vi "subCreateStagingPaths.vi"(0 "TestStand Version String":string="[2014, 2016, 2017]", 11 "error in":errorcluster) -> (3 "GACUtilityPaths":path[](array[path])=[path "C:/Users/admin/Documents/github/NIVeristandAdd-ons/VeriStand-steps-for-TestStand/Source/Source/CSharp/AddRemoveGACUtils/RemoveFromGAC.exe", path "C:/Users/admin/Documents/github/NIVeristandAdd-ons/VeriStand-steps-for-TestStand/Source/Source/CSharp/AddRemoveGACUtils/InstallToGAC.exe"], 4 "CSharp Assembly Project Path":path=path "C:/Users/admin/Documents/github/NIVeristandAdd-ons/VeriStand-steps-for-TestStand/Source/Source/CSharp/VeristandStepsAssembly/OpenWorkspaceDialog/VeristandSteps.csproj", 6 "TypePalette File Path":path=path "C:/Users/admin/Documents/github/NIVeristandAdd-ons/VeriStand-steps-for-TestStand/Source/Source/CustomPaletteFile/NI_VeristandTypes.ini", 8 "Program Files Destination Path":path=path "C:/Users/admin/Documents/github/NIVeristandAdd-ons/VeriStand-steps-for-TestStand/Source/Built/ProgramFiles_32/VeriStand Steps for TestStand", 10 "Icon File Path":path=path "C:/Users/admin/Documents/github/NIVeristandAdd-ons/VeriStand-steps-for-TestStand/Source/Source/CustomPaletteFile/Veristand_icon_vista.ico", 13 "Icon Paths":path[](array[path])=[path "C:/Users/admin/Documents/github/NIVeristandAdd-ons/VeriStand-steps-for-TestStand/Source/Built/documents/National Instruments/TestStand 2014 (32-bit)/Components/Icons", path "C:/Users/admin/Documents/github/NIVeristandAdd-ons/VeriStand-steps-for-TestStand/Source/Built/documents/National Instruments/TestStand 2014 (64-bit)/Components/Icons", path "C:/Users/admin/Documents/github/NIVeristandAdd-ons/VeriStand-steps-for-TestStand/Source/Built/documents/National Instruments/TestStand 2016 (32-bit)/Components/Icons", path "C:/Users/admin/Documents/github/NIVeristandAdd-ons/VeriStand-steps-for-TestStand/Source/Built/documents/National Instruments/TestStand 2016 (64-bit)/Components/Icons", path "C:/Users/admin/Documents/github/NIVeristandAdd-ons/VeriStand-steps-for-TestStand/Source/Built/documents/National Instruments/TestStand 2017 (32-bit)/Components/Icons", path "C:/Users/admin/Documents/github/NIVeristandAdd-ons/VeriStand-steps-for-TestStand/Source/Built/documents/National Instruments/TestStand 2017 (64-bit)/Components/Icons"], 14 "TypePalettes Paths":path[](array[path])=[path "C:/Users/admin/Documents/github/NIVeristandAdd-ons/VeriStand-steps-for-TestStand/Source/Built/documents/National Instruments/TestStand 2014 (32-bit)/Components/TypePalettes", path "C:/Users/admin/Documents/github/NIVeristandAdd-ons/VeriStand-steps-for-TestStand/Source/Built/documents/National Instruments/TestStand 2014 (64-bit)/Components/TypePalettes", path "C:/Users/admin/Documents/github/NIVeristandAdd-ons/VeriStand-steps-for-TestStand/Source/Built/documents/National Instruments/TestStand 2016 (32-bit)/Components/TypePalettes", path "C:/Users/admin/Documents/github/NIVeristandAdd-ons/VeriStand-steps-for-TestStand/Source/Built/documents/National Instruments/TestStand 2016 (64-bit)/Components/TypePalettes", path "C:/Users/admin/Documents/github/NIVeristandAdd-ons/VeriStand-steps-for-TestStand/Source/Built/documents/National Instruments/TestStand 2017 (32-bit)/Components/TypePalettes", path "C:/Users/admin/Documents/github/NIVeristandAdd-ons/VeriStand-steps-for-TestStand/Source/Built/documents/National Instruments/TestStand 2017 (64-bit)/Components/TypePalettes"], 15 "Error out":errorcluster)   [LabVIEW 2015]
uses:
  veristand-steps-build-tools.lvlib
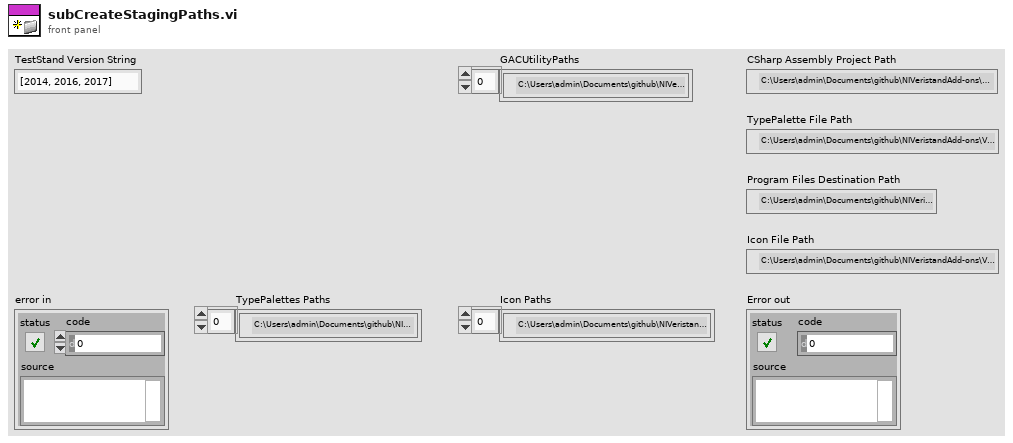
[diagram p1: front panel]
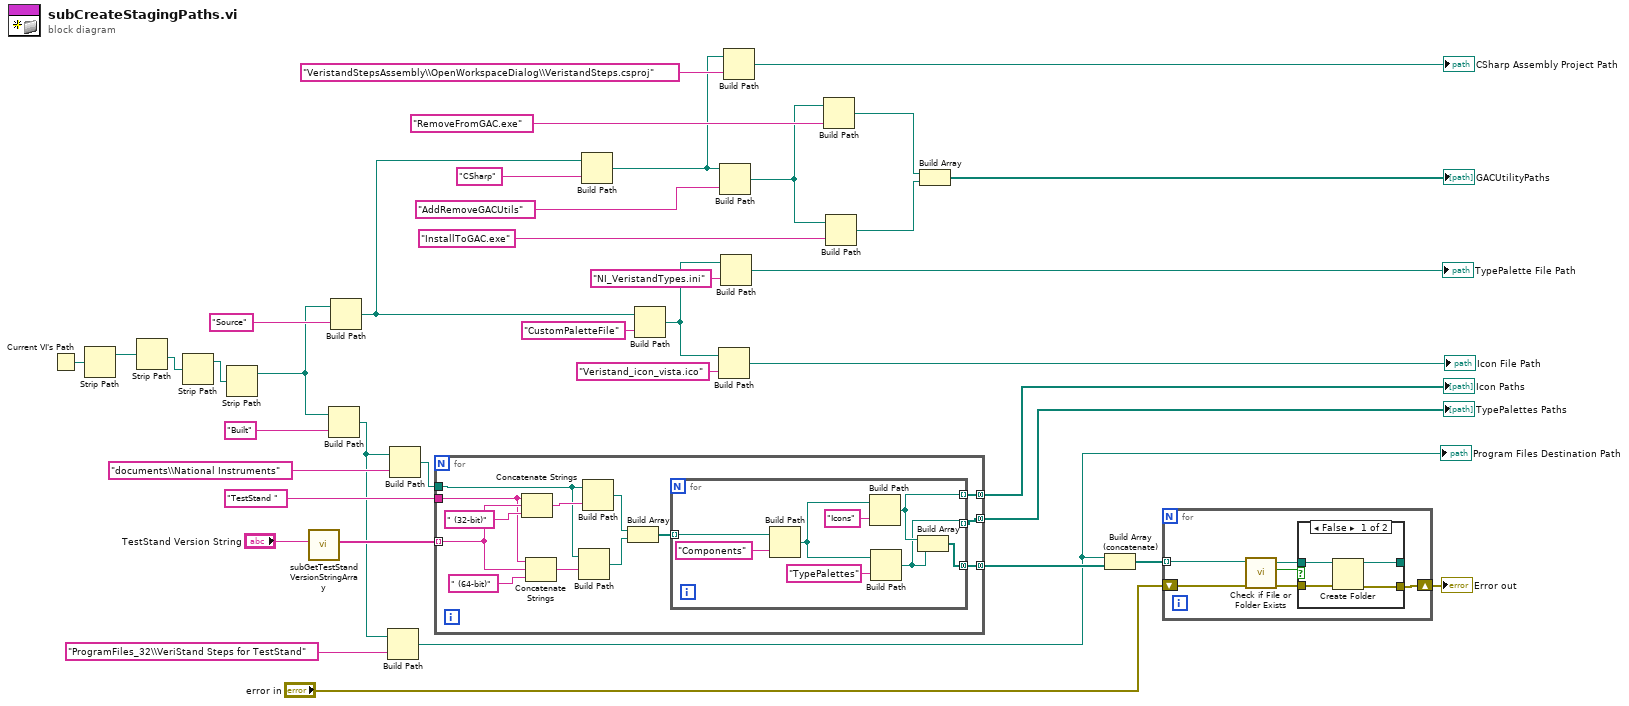
[diagram p0: block diagram]
diagram:
  n1 = Current VI's Path() -> (path=w31:path)
  n2 = Strip Path(path=w31) -> (stripped path=w30:path)  [unwired: 1 out]
  n3 = Strip Path(path=w30) -> (stripped path=w29:path)  [unwired: 1 out]
  n4 = Strip Path(path=w29) -> (stripped path=w2:path)  [unwired: 1 out]
  n5 = Strip Path(path=w2) -> (stripped path=w1:path)  [unwired: 1 out]
  n6 = call "subGetTestStandVersionStringArray.vi"("TestStand Version String"="TestStand Version String") -> ("TestStand Version String Array"=w37:string[])  [unwired: 10 in]
  n7 = Build Path(base path=w1, name or relative path="Built") -> (appended path=w28:path)
  n8 = Build Path(base path=w1, name or relative path="Source") -> (appended path=w11:path)
  n9 = Build Path(base path=w28, name or relative path="ProgramFiles_32\\VeriStand Steps for TestStand") -> (appended path=w13:path)
  "Program Files Destination Path" <- w13
  n10 = Build Path(base path=w28, name or relative path="documents\\National Instruments") -> (appended path=w14:path)
  n11 = for {
    tunnel: w37 -> [w50] mode=indexing
    tunnel: w14 -> [w47]
    tunnel: "TestStand " ("name or relative path") -> [w46]
    tunnel: [w42] -> w32 mode=concatenating
    tunnel: [w41] -> w19 mode=concatenating
    tunnel: [w40] -> w18 mode=concatenating
    n12 = Concatenate Strings(w46, w50, " (32-bit)" ("string")) -> (w48:string)
    n13 = Concatenate Strings(w46, w50, " (64-bit)" ("string")) -> (w49:string)
    n14 = Build Path(base path=w47, name or relative path=w49) -> (appended path=w44:path)
    n15 = Build Path(base path=w47, name or relative path=w48) -> (appended path=w45:path)
    n16 = Build Array(w45, w44) -> (w43:path[])
    n17 = for {
      tunnel: w43 -> [w60] mode=indexing
      tunnel: [w55] -> w42 mode=concatenating
      tunnel: [w54] -> w41 mode=indexing
      tunnel: [w53] -> w40 mode=indexing
      n18 = Build Path(base path=w60, name or relative path="Components") -> (appended path=w57:path)
      n19 = Build Path(base path=w57, name or relative path="Icons") -> (appended path=w54:path)
      n20 = Build Path(base path=w57, name or relative path="TypePalettes") -> (appended path=w53:path)
      n21 = Build Array(w54, w53) -> (w55:path[])
    }
  }
  "Icon Paths" <- w19
  "TypePalettes Paths" <- w18
  n22 = Build Path(base path=w11, name or relative path="CSharp") -> (appended path=w16:path)
  n23 = Build Path(base path=w11, name or relative path="CustomPaletteFile") -> (appended path=w9:path)
  n24 = Build Path(base path=w9, name or relative path="Veristand_icon_vista.ico") -> (appended path=→"Icon File Path":path)
  n25 = Build Path(base path=w16, name or relative path="AddRemoveGACUtils") -> (appended path=w22:path)
  n26 = Build Path(base path=w9, name or relative path="NI_VeristandTypes.ini") -> (appended path=→"TypePalette File Path":path)
  n27 = Build Path(base path=w16, name or relative path="VeristandStepsAssembly\\OpenWorkspaceDialog\\VeristandSteps.csproj") -> (appended path=→"CSharp Assembly Project Path":path)
  n28 = Build Path(base path=w22, name or relative path="RemoveFromGAC.exe") -> (appended path=w25:path)
  n29 = Build Path(base path=w22, name or relative path="InstallToGAC.exe") -> (appended path=w26:path)
  n30 = Build Array(w25, w26) -> (→"GACUtilityPaths":path[])
  n31 = Build Array (concatenate)(w13, w32) -> (w33:path[])
  n32 = for {
    shift-right: [w63] -> w3
    shift-left: "error in" -> [w62]
    tunnel: w33 -> [w61] mode=indexing
    n33 = call <vilib>:"Check if File or Folder Exists.vi"("error in (no error)"=w62, "path"=w61) -> ("error out"=w66:errorcluster, "file or folder exists?"=w64:bool, "dup path"=w65:path)  [unwired: 7 in]
    n34 = case shown="False" w64 {
      tunnel: w66 -> [w70 w71]
      tunnel: w65 -> [w69 w72]
      tunnel: [w68 w71] -> w63
      tunnel: [w67 w72] -> _
      frame False {
        n35 = Create Folder(path (use dialog)=w69, error in=w70) -> (created path=w67:path, error out=w68:errorcluster)  [unwired: 1 in, 1 out]
      }
      frame True {
      }
    }
  }
  "Error out" <- w3
